vi "FPGA_Q1_MODULE.vi"() -> ()   [LabVIEW 2018]
uses:
  <vilib>/rvi/Emulation/niFpgaGetClockAttributes.vi
  <vilib>/rvi/Emulation/niFpgaSctlEmulationGetInTimedLoop.vi
  <vilib>/rvi/Emulation/niFpgaEmulationReportErrorSimple.vi
  <vilib>/rvi/eio/common/nirviEmuTemplateMethod_errors.vi
  <vilib>/rvi/Emulation/niFpgaCriticalErrorInLSC.vi
  <vilib>/eio/EIONode/EIONode.xnode
panel:
  in  "Mod2/AO0":i16
  out "Mod2/AI0":i16
  out "Mod1/EI0 Index Position":i32
  out "Mod1/EI0 Position":i32
  out "Mod1/EI1 Index Position":i32
  out "Mod1/EI1 Position":i32
  out "Mod2/EI0 Index Position":i32
  out "Mod2/EI0 Position":i32
  out "Mod2/EI1 Index Position":i32
  out "Mod2/EI1 Position":i32
  out "Mod1/AI0":i16
  in  "Mod1/AO0":i16
  in  "stop":bool
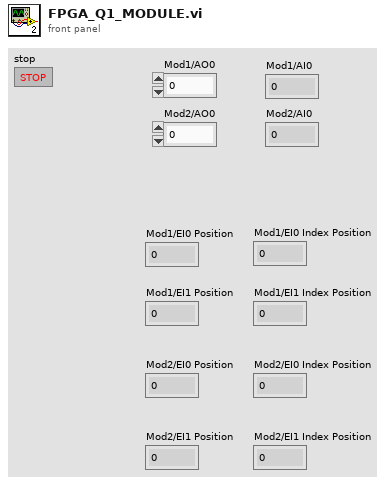
[diagram p1: front panel]
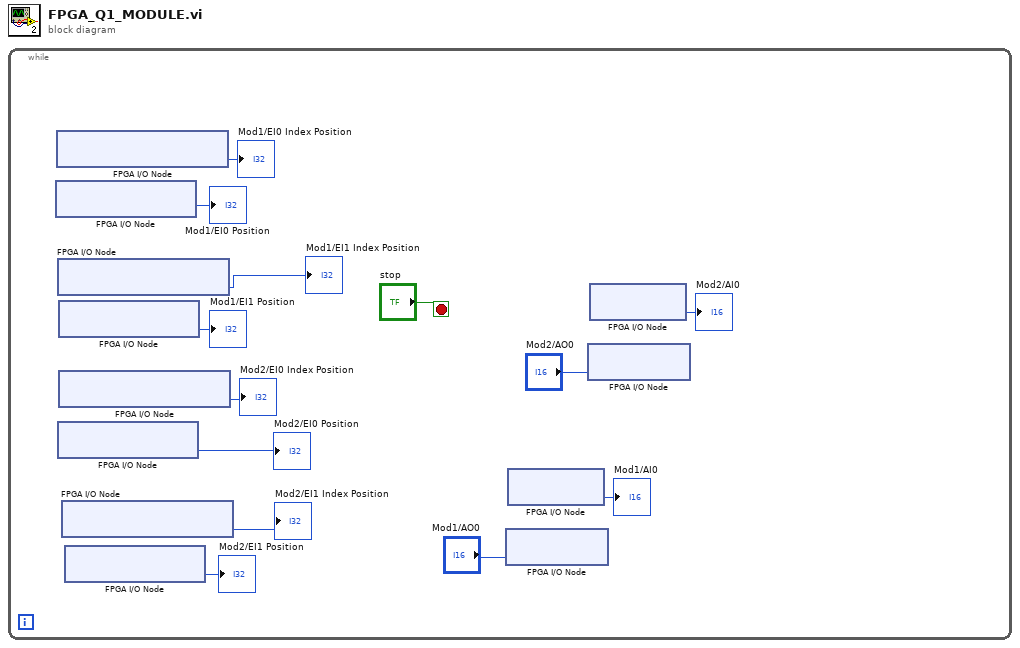
[diagram p0: block diagram]
diagram:
  n1 = while {
    stop <- "stop" stop-if-true
    n2 = xnode "FPGA I/O Node"() -> ("Mod1/EI0 Position"=→"Mod1/EI0 Position":i32)  [unwired: 1 in, 1 out]
    n3 = xnode "FPGA I/O Node"() -> ("Mod1/EI0 Index Position"=→"Mod1/EI0 Index Position":i32)  [unwired: 1 in, 1 out]
    n4 = xnode "FPGA I/O Node"() -> ("Mod1/EI1 Index Position"=→"Mod1/EI1 Index Position":i32)  [unwired: 1 in, 1 out]
    n5 = xnode "FPGA I/O Node"() -> ("Mod2/EI0 Position"=→"Mod2/EI0 Position":i32)  [unwired: 1 in, 1 out]
    n6 = xnode "FPGA I/O Node"() -> ("Mod1/EI1 Position"=→"Mod1/EI1 Position":i32)  [unwired: 1 in, 1 out]
    n7 = xnode "FPGA I/O Node"() -> ("Mod2/EI0 Index Position"=→"Mod2/EI0 Index Position":i32)  [unwired: 1 in, 1 out]
    n8 = xnode "FPGA I/O Node"() -> ("Mod2/EI1 Index Position"=→"Mod2/EI1 Index Position":i32)  [unwired: 1 in, 1 out]
    n9 = xnode "FPGA I/O Node"() -> ("Mod2/EI1 Position"=→"Mod2/EI1 Position":i32)  [unwired: 1 in, 1 out]
    n10 = xnode "FPGA I/O Node"("Mod1/AO0"="Mod1/AO0") -> ()  [unwired: 1 in, 1 out]
    n11 = xnode "FPGA I/O Node"() -> ("Mod1/AI0"=→"Mod1/AI0":i16)  [unwired: 1 in, 1 out]
    n12 = xnode "FPGA I/O Node"("Mod2/AO0"="Mod2/AO0") -> ()  [unwired: 1 in, 1 out]
    n13 = xnode "FPGA I/O Node"() -> ("Mod2/AI0"=→"Mod2/AI0":i16)  [unwired: 1 in, 1 out]
  }
